vi "open-camera-file.vi"(10 "file_format":i32, 11 "filename":path) -> (3 "ir_file_handler":u64)   [LabVIEW 2011, in "librir.lvlib"]
uses:
  librir.lvlib
  libs/video_io.dll
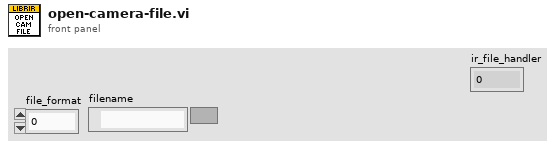
[diagram p1: front panel]
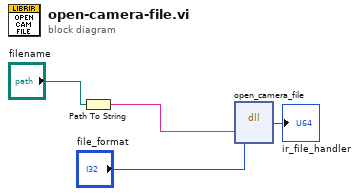
[diagram p0: block diagram]
diagram:
  n1 = Path To String(path="filename") -> (string=w1:string)
  n2 = dll-call lib="G:/librir/src/labview/libs/video_io.dll" fn="open_camera_file"("filename"=w1, "file_format"="file_format") -> ("ir_file_handler"=→"ir_file_handler":u64)  [unwired: 5 in, 2 out]
